vi "Untitled 4 (SubVI).vi"(0 "Position Reset":bool, 1 "Radius of motor pulley\n (mm)":dbl, 5 "Length of the FCM (m)":dbl, 7 "Radius of disk (m)":dbl, 9 "Number of Disks":dbl, 12 "Tip position Input":dbl[](array[numeric])) -> (2 "L1 (m)":dbl, 3 "L2 (m)":dbl, 4 "L3 (m)":dbl, 6 "theta1":dbl, 8 "theta2":dbl, 10 "theta3":dbl, 13 "L_v":dbl, 14 "alpha":dbl, 15 "error out":errorcluster)   [LabVIEW 2019]
uses:
  <vilib>/imath/engines/lvmath2/RunTimeEngine/Managers/WorkSpace/UID Generator.vi
  <vilib>/imath/engines/lvmath2/RunTimeEngine/IndexRead/NIMS V(S).vi
  <instcachedir>/0/NIMS V(S)_0488751826AF41519A22953C041130DC.lvgen/NIMS V(S)_0488751826AF41519A22953C041130DC_000.vi
  <vilib>/imath/engines/lvmath2/RunTimeEngine/BuiltInFunctions/atan2/NIMS_atan2.vi
  <instcachedir>/0/NIMS_atan2_A91AA4A7D42247EDBE8F76DB99AF04A4.lvgen/NIMS_atan2_A91AA4A7D42247EDBE8F76DB99AF04A4_000.vi
  <vilib>/imath/engines/lvmath2/RunTimeEngine/RunTimeType/NIMS_RunTimeType_From StrictType (excl LVString).vi
  <instcachedir>/0/NIMS_RunTimeType_From StrictType (excl LVString)_D8AFBA86A94845AAA577C895450664BD.lvgen/NIMS_RunTimeType_From StrictType (excl LVString)_D8AFBA86A94845AAA577C895450664BD_000.vi
  <vilib>/imath/engines/lvmath2/RunTimeEngine/ErrorHandling/NIMS_Create Error From Enums.vi
  <vilib>/imath/engines/lvmath2/RunTimeEngine/LocalVariableDefStatement/MC_LocalVariableDefStatement_Display.vi
  <vilib>/imath/engines/lvmath2/RunTimeEngine/BuiltInFunctions/atan/NIMS_atan(C).vi
  <instcachedir>/0/NIMS_atan(C)_0A85D365582D4E8AB3874BC9125E138E.lvgen/NIMS_atan(C)_0A85D365582D4E8AB3874BC9125E138E_001.vi
  <vilib>/imath/engines/lvmath2/RunTimeEngine/BuiltInFunctions/cross/NIMS_cross(GV,GV).vi
  <instcachedir>/0/NIMS_cross(GV,GV)_6F1F1C643EFF41C8A983D972A94A5A15.lvgen/NIMS_cross(GV,GV)_6F1F1C643EFF41C8A983D972A94A5A15_000.vi
  <vilib>/imath/engines/lvmath2/RunTimeEngine/BuiltInFunctions/norm/NIMS_norm(GV,DBL).vi
  <instcachedir>/0/NIMS_norm(GV,DBL)_4A8B6F23BC0A47549B8AB805006257D9.lvgen/NIMS_norm(GV,DBL)_4A8B6F23BC0A47549B8AB805006257D9_000.vi
  <vilib>/imath/engines/lvmath2/RunTimeEngine/ArithmeticOperatorToken/NIMS_ArithmeticOperator_multmx-internal.vi
  <instcachedir>/0/NIMS_ArithmeticOperator_multmx-internal_9E91BA3A2DCB4083AAD724A04442A6F7.lvgen/NIMS_ArithmeticOperator_multmx-internal_9E91BA3A2DCB4083AAD724A04442A6F7_004.vi
  <vilib>/imath/engines/lvmath2/RunTimeEngine/BuiltInFunctions/cos/NIMS_cos(C).vi
  <instcachedir>/0/NIMS_cos(C)_BED070B05FDB4939A63CB05E18805866.lvgen/NIMS_cos(C)_BED070B05FDB4939A63CB05E18805866_001.vi
  <vilib>/imath/engines/lvmath2/RunTimeEngine/BuiltInFunctions/sin/NIMS_sin(C).vi
  <instcachedir>/0/NIMS_sin(C)_6504C6AC704B4661870B0E93397B11C4.lvgen/NIMS_sin(C)_6504C6AC704B4661870B0E93397B11C4_001.vi
  <vilib>/imathl/engines/lvmath/Functions/Error Handling/Create Error.vi
  <vilib>/imath/engines/lvmath2/RunTimeEngine/ArithmeticOperatorToken/NIMS_ArithmeticOperator_multmx(M,CV)-internal.vi
  <instcachedir>/0/NIMS_ArithmeticOperator_multmx(M,CV)-internal_2C55777844884EEDB828A940D397C7D0.lvgen/NIMS_ArithmeticOperator_multmx(M,CV)-internal_2C55777844884EEDB828A940D397C7D0_002.vi
  <instcachedir>/0/NIMS_norm(GV,DBL)_4A8B6F23BC0A47549B8AB805006257D9.lvgen/NIMS_norm(GV,DBL)_4A8B6F23BC0A47549B8AB805006257D9_001.vi
  <vilib>/imath/engines/lvmath2/RunTimeEngine/Managers/SymbolTable/Clear UID.vi
  <vilib>/imath/engines/lvmath2/RunTimeEngine/NodeEndStatement/NIMS_NodeEndStatement_Output.vi
  <instcachedir>/0/NIMS_NodeEndStatement_Output_53EC0D466D134D7ABD903AC30B43404B.lvgen/NIMS_NodeEndStatement_Output_53EC0D466D134D7ABD903AC30B43404B_001.vi
  <vilib>/imath/engines/lvmath2/RunTimeEngine/ErrorHandling/NIMS_Finalize Error.vi
  <vilib>/imath/engines/lvmath2/RunTimeEngine/Managers/SymbolTable/NIMS_WorkSpace.lvlib
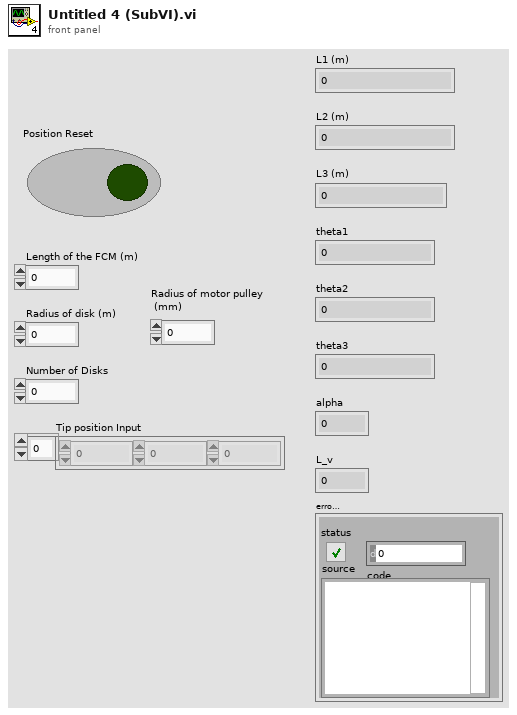
[diagram p1: front panel]
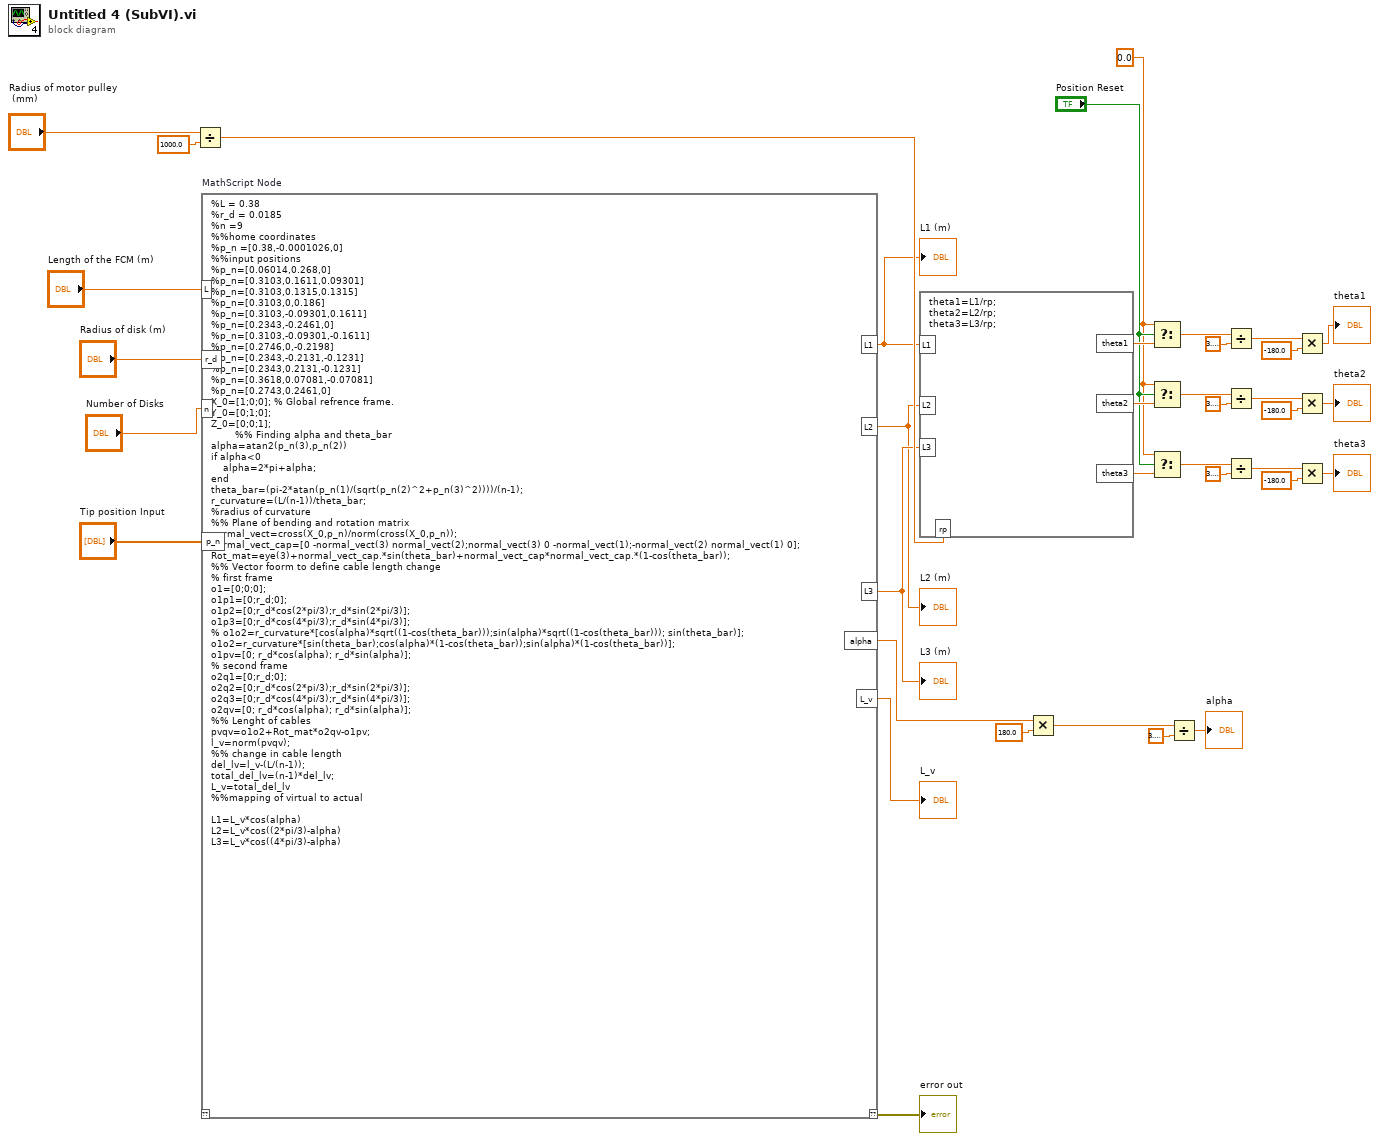
[diagram p0: block diagram]
diagram:
  w13 = 0.0 ("t")
  n1 = Divide(x="Radius of motor pulley\n (mm)", y=1000.0) -> (x/y=w31:dbl)
  n2 = mathscript code="%L = 0.38\n%r_d = 0.0185\n%n =9 \n%%home coordinates\n%p_n =[0.38,-0.0001026,0] \n%%input positions\n%p_n=[0.06014,0.268,0]\n%p_n=[0.3103,0.1611,0.09301]\n%p_n=[0.3103,0.1315,0.1315]\n%p_n=[0.3103,0,0.186]\n%p_n=[0.3103,-0.09301,0.1611]\n%p_n=[0.2343,-0.2461,0]\n%p_n=[0.3103,-0.09301,-0.1611]\n%p_n=[0.2746,0,-0.2198]\n%p_n=[0.2343,-0.2131,-0.1231]\n%p_n=[0.2343,0.2131,-0.1231]\n%p_n=[0.3618,0.07081,-0.07081]\n%p_n=[0.2743,0.2461,0]\nX_0=[1;0;0]; % Global refrence frame.\nY_0=[0;1;0];\nZ_0=[0;0;1];\n        %% Finding alpha and theta_bar\nalpha=atan2(p_n(3),p_n(2))\nif alpha<0\n    alpha=2*pi+alpha;\nend\ntheta_bar=(pi-2*atan(p_n(1)/(sqrt(p_n(2)^2+p_n(3)^2))))/(n-1);\nr_curvature=(L/(n-1))/theta_bar; \n%radius of curvature\n%% Plane of bending and rotation matrix\nnormal_vect=cross(X_0,p_n)/norm(cross(X_0,p_n));\nnormal_vect_cap=[0 -normal_vect(3) normal_vect(2);normal_vect(3) 0 -normal_vect(1);-normal_vect(2) normal_vect(1) 0];\nRot_mat=eye(3)+normal_vect_cap.*sin(theta_bar)+normal_vect_cap*normal_vect_cap.*(1-cos(theta_bar));\n%% Vector foorm to define cable length change\n% first frame\no1=[0;0;0];\no1p1=[0;r_d;0];\no1p2=[0;r_d*cos(2*pi/3);r_d*sin(2*pi/3)];\no1p3=[0;r_d*cos(4*pi/3);r_d*sin(4*pi/3)];\n% o1o2=r_curvature*[cos(alpha)*sqrt((1-cos(theta_bar)));sin(alpha)*sqrt((1-cos(theta_bar))); sin(theta_bar)];\no1o2=r_curvature*[sin(theta_bar);cos(alpha)*(1-cos(theta_bar));sin(alpha)*(1-cos(theta_bar))];\no1pv=[0; r_d*cos(alpha); r_d*sin(alpha)];\n% second frame\no2q1=[0;r_d;0];\no2q2=[0;r_d*cos(2*pi/3);r_d*sin(2*pi/3)];\no2q3=[0;r_d*cos(4*pi/3);r_d*sin(4*pi/3)];\no2qv=[0; r_d*cos(alpha); r_d*sin(alpha)];\n%% Lenght of cables\npvqv=o1o2+Rot_mat*o2qv-o1pv;\nl_v=norm(pvqv);\n%% change in cable length\ndel_lv=l_v-(L/(n-1));\ntotal_del_lv=(n-1)*del_lv;\nL_v=total_del_lv\n%%mapping of virtual to actual\n\nL1=L_v*cos(alpha)\nL2=L_v*cos((2*pi/3)-alpha)\nL3=L_v*cos((4*pi/3)-alpha)"("L"="Length of the FCM (m)", "r_d"="Radius of disk (m)", "n"="Number of Disks", "p_n"="Tip position Input") -> ("??"=→"error out":errorcluster, "L1"=w10:dbl, "L2"=w9:dbl, "L3"=w11:dbl, "alpha"=w8:dbl, "L_v"=→"L_v":dbl)  [unwired: 1 in]
  "L1 (m)" <- w10
  "L2 (m)" <- w9
  "L3 (m)" <- w11
  n3 = formula code="theta1=L1/rp;\ntheta2=L2/rp;\ntheta3=L3/rp;"("L1"=w10, "L2"=w9, "L3"=w11, "rp"=w31) -> ("theta1"=w19:dbl, "theta2"=w36:dbl, "theta3"=w15:dbl)
  n4 = Multiply(x=w8, y=180.0) -> (x*y=w6:dbl)
  n5 = Select(t=w13, s="Position Reset", f=w19) -> (s? t:f=w18:dbl)
  n6 = Select(t=w13, s="Position Reset", f=w36) -> (s? t:f=w17:dbl)
  n7 = Select(t=w13, s="Position Reset", f=w15) -> (s? t:f=w16:dbl)
  n8 = Divide(x=w6, y=3.141592653589793) -> (x/y=→"alpha":dbl)
  n9 = Divide(x=w18, y=3.141592653589793) -> (x/y=w27:dbl)
  n10 = Divide(x=w17, y=3.141592653589793) -> (x/y=w24:dbl)
  n11 = Divide(x=w16, y=3.141592653589793) -> (x/y=w21:dbl)
  n12 = Multiply(x=w27, y=-180.0) -> (x*y=→"theta1":dbl)
  n13 = Multiply(x=w24, y=-180.0) -> (x*y=→"theta2":dbl)
  n14 = Multiply(x=w21, y=-180.0) -> (x*y=→"theta3":dbl)
